vi "_StripCotentTag.vi"(11 "XML String":string="<ObjXMLNode>\r\n  <ModuleName>WaveformGen</ModuleName>\r\n  <ObjName>WaveformGen</ObjName>\r<Terminal Name=\"WaveformGen.Waveform\" TerminalType=\"Output\">\r<ObjXMLNode>\r\n  <ModuleName>WaveformDisplay</ModuleName>\r\n  <ObjName>Display1</ObjName>\r\n</ObjXMLNode>\r<ObjXMLNode>\r\n  <ModuleName>WaveformStreaming</ModuleName>\r\n  <ObjName>Streaming</ObjName>\r\n</ObjXMLNode>\r<ObjXMLNode>\r\n  <ModuleName>WaveformFFT</ModuleName>\r\n  <ObjName>WaveformFFT</ObjName>\r<Terminal Name=\"WaveformFFT.FFT\" TerminalType=\"Output\">\r<ObjXMLNode>\r\n  <ModuleName>WaveformDisplay</ModuleName>\r\n  <ObjName>Display3</ObjName>\r\n</ObjXMLNode>\r</Terminal>\r</ObjXMLNode>\r<ObjXMLNode>\r\n  <ModuleName>WaveformHistoryCache</ModuleName>\r\n  <ObjName>WaveformHistoryCache</ObjName>\r<Terminal Name=\"WaveformHistoryCache.HistoryCache\" TerminalType=\"Output\">\r<ObjXMLNode>\r\n  <ModuleName>WaveformDisplay</ModuleName>\r\n  <ObjName>Display2</ObjName>\r\n</ObjXMLNode>\r</Terminal>\r</ObjXMLNode>\r</Terminal>\r</ObjXMLNode>") -> (3 "delimited string":string)   [LabVIEW 2017]
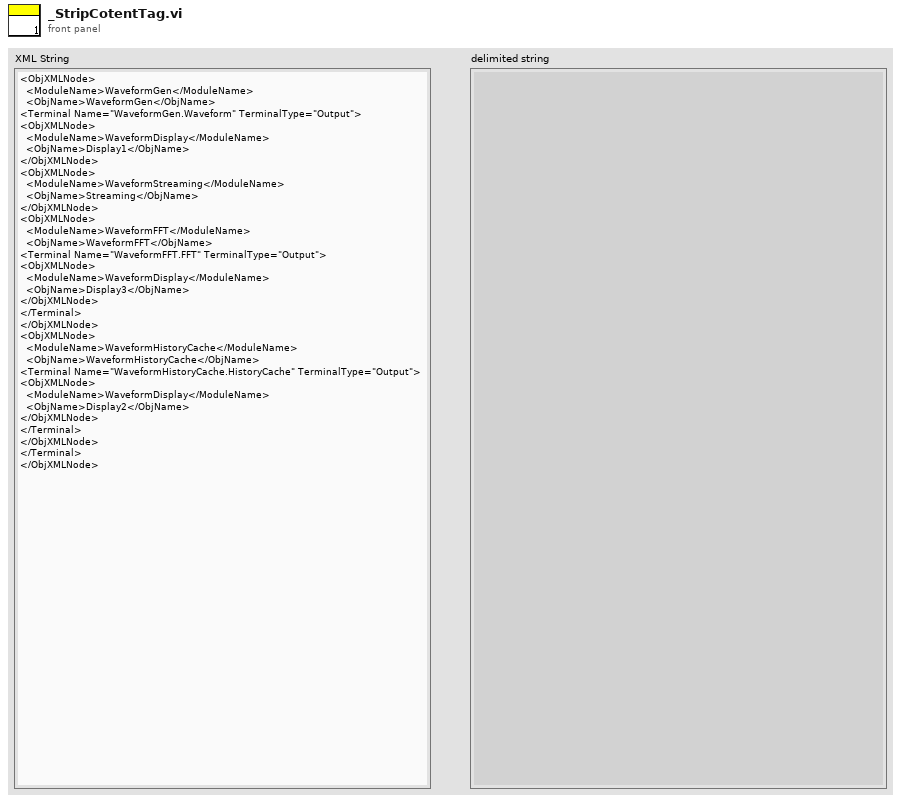
[diagram p1: front panel]
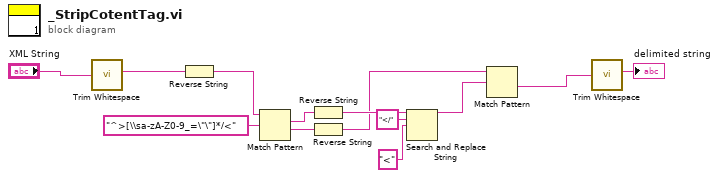
[diagram p0: block diagram]
diagram:
  n1 = call <vilib>:"Trim Whitespace.vi"("string"="XML String") -> ("trimmed string"=w1:string)  [unwired: 1 in]
  n2 = Reverse String(1:w1) -> (0:w9:string)
  n3 = Match Pattern(string=w9, regular expression="^>[\\sa-zA-Z0-9_=\"\"]*/<" ("string")) -> (match substring=w10:string, after substring=w11:string)  [unwired: 1 in, 2 out]
  n4 = Reverse String(1:w10) -> (0:w7:string)
  n5 = Reverse String(1:w11) -> (0:w4:string)
  n6 = Search and Replace String(input string=w7, search string="</", replace string="<" ("search string")) -> (result string=w3:string)  [unwired: 5 in, 3 out]
  n7 = Match Pattern(string=w4, regular expression=w3) -> (after substring=w13:string)  [unwired: 1 in, 3 out]
  n8 = call <vilib>:"Trim Whitespace.vi"("string"=w13) -> ("trimmed string"=→"delimited string":string)  [unwired: 1 in]
